vi "DataAcquisition.vi"() -> ()   [LabVIEW 2021]
uses:
  <instrlib>/niDMM/nidmm.llb/niDMM Function.ctl
  <instrlib>/niDMM/nidmm.llb/niDMM Configure Measurement Absolute.vi
  <instrlib>/niSwitch/niSwitch.llb/niSwitch Connect Channels (Single).vi
  <vilib>/express/express analysis/Spectral/Block/exnSpectralBlock spectral measurements RMS poly.vi
  <vilib>/express/express analysis/Spectral/Block/exnSpectralBlock spectral measurements RMS DDT.vi
  <vilib>/express/express analysis/Spectral/XNode/ExpressSpectralMeasurementsBlockNode.xnode
panel:
  out "Spectral Analysis: Magnitude":dynamicdata(graph)
  in  "Number Of Drops":dbl
  in  "Path":path
  out "2nd Trigger":bool
  out "1st Trigger":bool
  out "Spectral Analysis: Phase":dynamicdata(graph)
  out "Time Series":dynamicdata(graph)
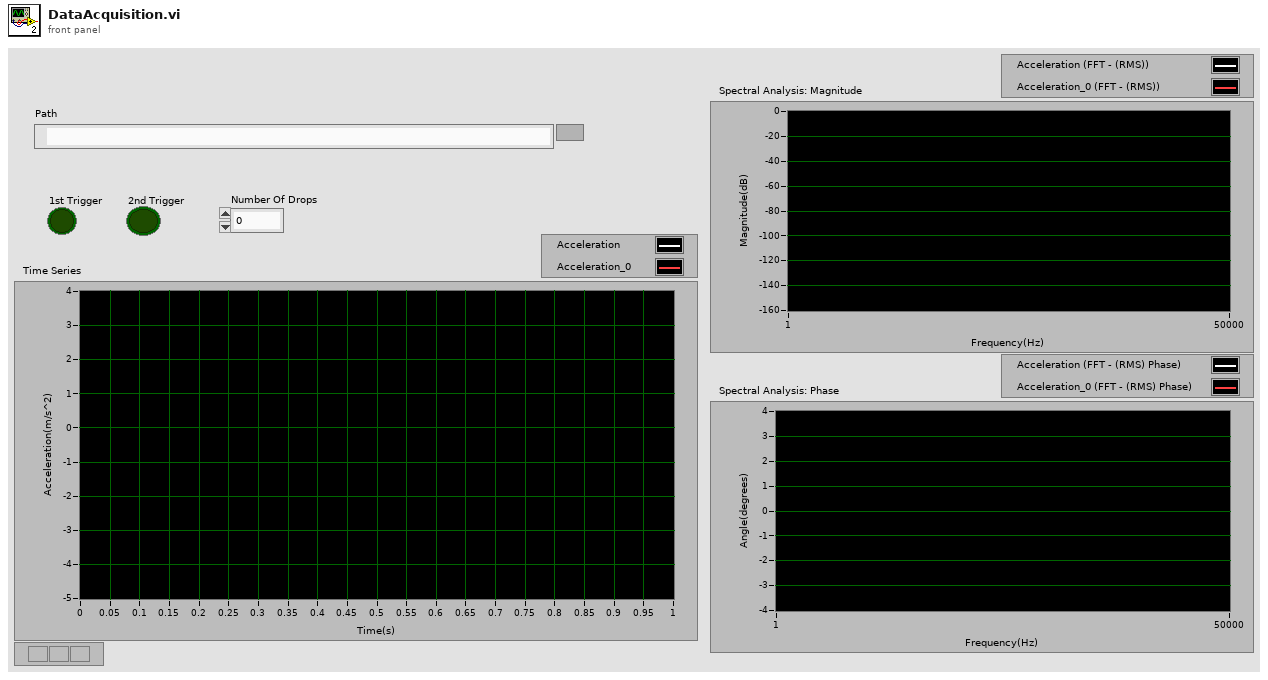
[diagram p1: front panel]
types:
  T1 = typedef "niDMM Function.ctl" = enum16{"DC Volts", "AC Volts", "DC Current", "AC Current", "2-wire Resistance", "4-wire Resistance", "Diode", "Frequency", "Period", "AC Volts DC Coupled", "Capacitance", "Inductance", "Temperature"}
  T2 = enum16{"open", "replace", "create", "open or create", "replace or create", "replace or create with confirmation"}
  T3 = cluster{"averaging mode":u16, "weighting mode":u16, "number of averages":u32}
  T4 = cluster{"dB On (F)":bool, "unwrap phase (F)":bool, "convert to degree (F)":bool}
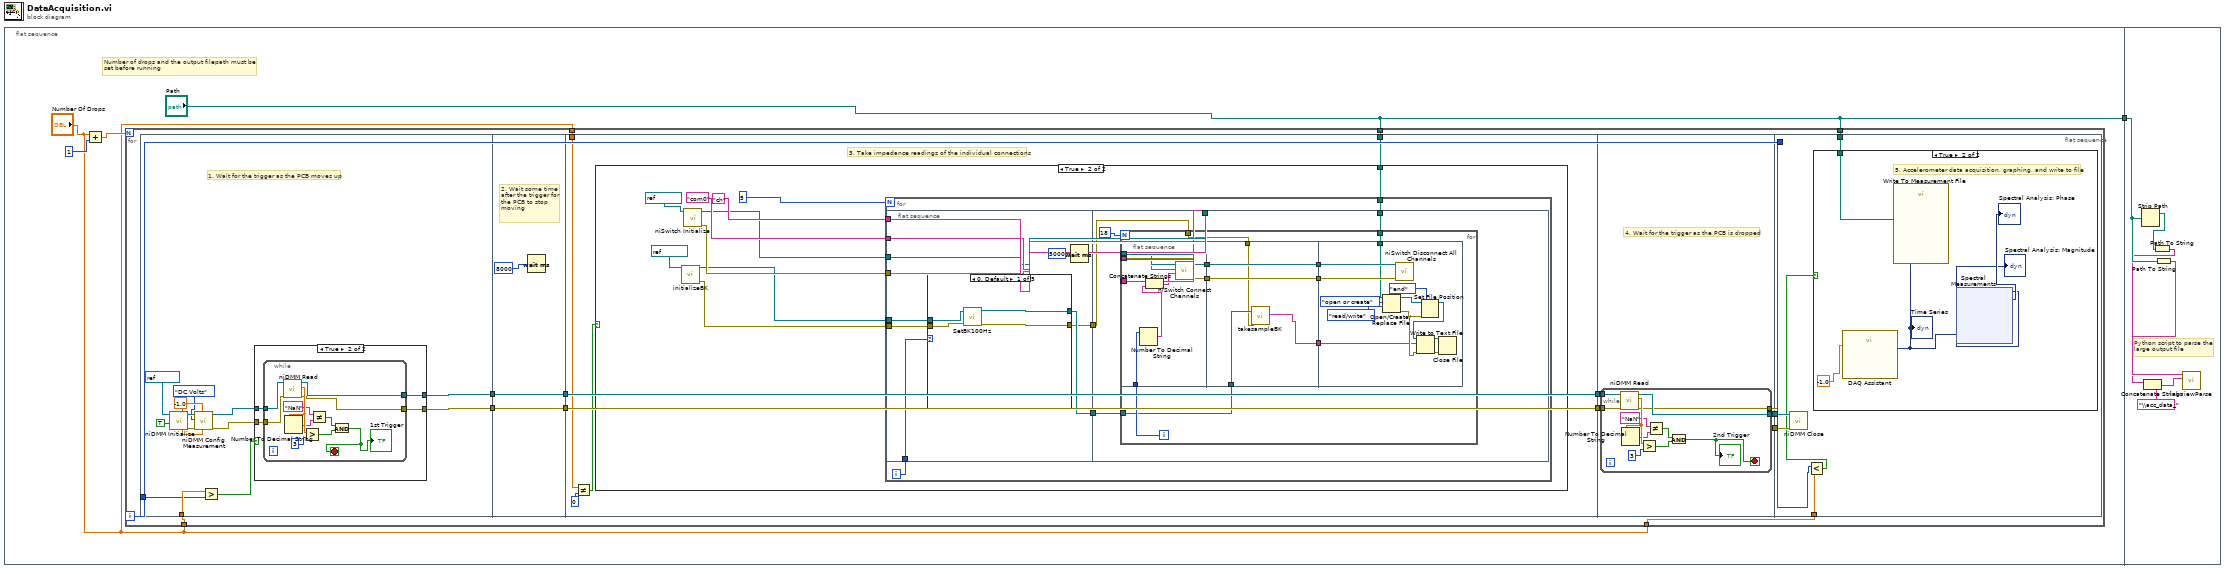
[diagram p0: block diagram]
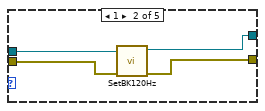
[diagram p4: hidden frame]
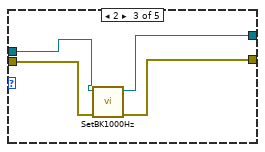
[diagram p5: hidden frame]
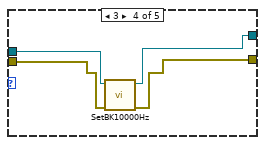
[diagram p6: hidden frame]
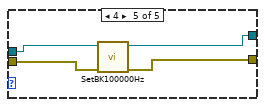
[diagram p7: hidden frame]
diagram:
  n1 = flat-sequence {
    tunnel: ["Path"] -> w1
    tunnel: w1 -> [w193]
    frame #0 {
      # "Number of drops and the output filepath must be\nset before running"
      n2 = Add(x="Number Of Drops", y=1) -> (x+y=w4:dbl)
      n3 = for {
        N: w4 -> [_]
        tunnel: "Number Of Drops" -> [w15]
        tunnel: "Number Of Drops" -> [w14]
        tunnel: "Path" -> [w8]
        tunnel: "Number Of Drops" -> [w7]
        tunnel: "Path" -> [w6]
        i -> [w13]
        n4 = flat-sequence {
          tunnel: [w24] -> w12
          tunnel: [w23] -> w10
          tunnel: w14 -> [w22]
          tunnel: w13 -> [w21]
          tunnel: w12 -> [w52]
          tunnel: [w52] -> w11
          tunnel: w10 -> [w51]
          tunnel: [w51] -> w9
          tunnel: [w58] -> w19
          tunnel: w11 -> [w58]
          tunnel: [w57] -> w18
          tunnel: w9 -> [w57]
          tunnel: w7 -> [w55]
          tunnel: w6 -> [w53]
          tunnel: w19 -> [w156]
          tunnel: w18 -> [w155]
          tunnel: [w154] -> w17
          tunnel: [w153] -> w16
          tunnel: w17 -> [w173]
          tunnel: w16 -> [w172]
          tunnel: w13 -> [w171]
          tunnel: w15 -> [w170]
          tunnel: w8 -> [w168]
          frame #0 {
            w27 = -1.0
            # "1. Wait for the trigger as the PCB moves up"
            n5 = call <instrlib>:"niDMM Initialize.vi"("Reset"=TRUE, "Instrument Descriptor"=refnum<k15> "DMM") -> ("error out"=w29:errorcluster, "instrument handle out"=w30:refnum<k15>)  [unwired: 8 in]
            n6 = call-poly <instrlib>:"niDMM Config Measurement.vi"("Range"=w27, "Resolution"=w27, "error in (no error)"=w29, "Function"=niDMM_Function."DC Volts", "instrument handle"=w30) -> ("error out"=w32:errorcluster, "instrument handle out"=w31:refnum<k15>)  [unwired: 5 in]
            n7 = Greater?(x=w22, y=w21) -> (0:w20:bool)
            n8 = case shown="True" w20 {
              tunnel: w32 -> [w34 w38]
              tunnel: w31 -> [w33 w37]
              tunnel: [w33 w36] -> w24
              tunnel: [w34 w35] -> w23
              frame False {
              }
              frame True {
                n9 = while {
                  tunnel: w37 -> [w49]
                  tunnel: w38 -> [w48]
                  tunnel: [w41] -> w36
                  tunnel: [w40] -> w35
                  stop <- w39 stop-if-true
                  n10 = call <instrlib>:"niDMM Read.vi"("error in (no error)"=w48, "instrument handle"=w49) -> ("error out"=w40:errorcluster, "Measurement"=w46:dbl, "instrument handle out"=w41:refnum<k15>)  [unwired: 7 in]
                  n11 = Number To Decimal String(number=w46) -> (decimal integer string=w44:string)  [unwired: 1 in]
                  n12 = Greater?(x=w46, y=3) -> (0:w42:bool)
                  n13 = Not Equal?(x="NaN", y=w44) -> (x != y?=w43:bool)
                  n14 = And(x=w43, y=w42) -> (x .and. y?=w39:bool)
                  "1st Trigger" <- w39
                }
              }
            }
          }
          frame #1 {
            # "2. Wait some time\nafter the trigger for the PCB to stop moving"
            n15 = Wait (ms)(milliseconds to wait=u32 8000) -> ()  [unwired: 1 out]
          }
          frame #2 {
            # "3. Take impedance readings of the individual connections"
            n16 = Not Equal?(x=w55, y=0) -> (x != y?=w54:bool)
            n17 = case shown="True" w54 {
              tunnel: w53 -> [_ w59]
              frame False {
              }
              frame True {
                n18 = call "initializeBK.vi"("VISA resource name"=refnum<visa-resource-name> "COM7") -> ("error out"=w60:errorcluster, "VISA resource name out"=w61:refnum<visa-resource-name>)  [unwired: 8 in, 1 out]
                n19 = call <instrlib>:"niSwitch Initialize.vi"("resource name"=refnum<k15> "switch") -> ("error out"=w64:errorcluster, "instrument handle out"=w63:refnum<k15>)  [unwired: 9 in]
                n20 = for {
                  N: 5 -> [_]
                  tunnel: "ch" -> [w79]
                  tunnel: "com0" -> [w78]
                  tunnel: w64 -> [w77]
                  tunnel: w63 -> [w76]
                  tunnel: w61 -> [w74]
                  tunnel: w60 -> [w73]
                  tunnel: w59 -> [w70]
                  i -> [w75]
                  n21 = flat-sequence {
                    tunnel: w75 -> [w84]
                    tunnel: w74 -> [w83]
                    tunnel: w73 -> [w82]
                    tunnel: [w81] -> w72
                    tunnel: [w80] -> w71
                    tunnel: w79 -> [w112]
                    tunnel: w78 -> [w111]
                    tunnel: w77 -> [w110]
                    tunnel: w76 -> [w109]
                    tunnel: w72 -> [w107]
                    tunnel: w71 -> [w106]
                    tunnel: w70 -> [w105]
                    frame #0 {
                      n22 = case shown="0, Default" w84 {
                        tunnel: w83 -> [w88 w92 w96 w100 w104]
                        tunnel: w82 -> [w87 w91 w95 w99 w101]
                        tunnel: [w86 w90 w93 w97 w103] -> w81
                        tunnel: [w85 w89 w94 w98 w102] -> w80
                        frame 0, Default {
                          n23 = call "SetBK100Hz.vi"("error out 2"=w87, "VISA resource name out"=w88) -> ("error out"=w85:errorcluster, "VISA resource name out 2"=w86:refnum<visa-resource-name>)  [unwired: 5 in]
                        }
                        frame 1 {
                          n24 = call "SetBK120Hz.vi"("error out 2"=w91, "VISA resource name out"=w92) -> ("error out"=w89:errorcluster, "VISA resource name out 2"=w90:refnum<visa-resource-name>)  [unwired: 8 in]
                        }
                        frame 2 {
                          n25 = call "SetBK1000Hz.vi"("VISA resource name out"=w96, "error out 2"=w95) -> ("VISA resource name out 2"=w93:refnum<visa-resource-name>, "error out"=w94:errorcluster)  [unwired: 7 in]
                        }
                        frame 3 {
                          n26 = call "SetBK10000Hz.vi"("VISA resource name out"=w100, "error out 2"=w99) -> ("VISA resource name out 2"=w97:refnum<visa-resource-name>, "error out"=w98:errorcluster)  [unwired: 6 in]
                        }
                        frame 4 {
                          n27 = call "SetBK100000Hz.vi"("error out 2"=w101, "VISA resource name out"=w104) -> ("error out"=w102:errorcluster, "VISA resource name out 2"=w103:refnum<visa-resource-name>)  [unwired: 8 in]
                        }
                      }
                    }
                    frame #1 {
                      n28 = for {
                        N: 18 -> [_]
                        tunnel: w112 -> [w120]
                        tunnel: w111 -> [w119]
                        tunnel: w110 -> [w118]
                        tunnel: w109 -> [w117]
                        tunnel: w107 -> [w116]
                        tunnel: w106 -> [w115]
                        tunnel: w105 -> [w113]
                        i -> [w121]
                        n29 = flat-sequence {
                          tunnel: w117 -> [w134]
                          tunnel: w118 -> [w133]
                          tunnel: w119 -> [w132]
                          tunnel: [w131] -> w124
                          tunnel: [w130] -> w122
                          tunnel: w121 -> [w129]
                          tunnel: w120 -> [w126]
                          tunnel: [w139] -> w125
                          tunnel: w124 -> [w139]
                          tunnel: [w138] -> w123
                          tunnel: w122 -> [w138]
                          tunnel: w116 -> [w137]
                          tunnel: w115 -> [w136]
                          tunnel: [w135] -> w114
                          tunnel: w125 -> [w152]
                          tunnel: w123 -> [w151]
                          tunnel: w114 -> [w146]
                          tunnel: w113 -> [w140]
                          frame #0 {
                            n30 = Number To Decimal String(number=w129) -> (decimal integer string=w127:string)  [unwired: 1 in]
                            n31 = Concatenate Strings(w126, w127) -> (w128:string)
                            n32 = call-poly <instrlib>:"niSwitch Connect Channels.vi"("error in (no error)"=w133, "channel 2"=w128, "channel 1"=w132, "instrument handle"=w134) -> ("error out"=w130:errorcluster, "instrument handle out"=w131:refnum<k15>)  [unwired: 6 in]
                          }
                          frame #1 {
                            n33 = call "takesampleBK.vi"("error in (no error)"=w136, "VISA resource name"=w137) -> ("current sample"=w135:string)  [unwired: 7 in, 2 out]
                          }
                          frame #2 {
                            n34 = Open/Create/Replace File(file path (use dialog)=w140, operation (0:open)=T2."open or create", access (0:read/write)=enum16{"read/write", "read-only", "write-only"}."read/write") -> (refnum out=w150:refnum<file>, error out=w149:errorcluster)  [unwired: 3 in, 1 out]
                            n35 = call <instrlib>:"niSwitch Disconnect All Channels.vi"("error in (no error)"=w151, "instrument handle"=w152) -> ()  [unwired: 8 in, 2 out]
                            n36 = Set File Position(refnum=w150, from (0:start)=enum16{"start", "end", "current"}."end", error in=w149) -> (refnum out=w148:refnum<file>, error out=w147:errorcluster)  [unwired: 1 in]
                            n37 = Write to Text File(file (use dialog)=w148, text=w146, error in=w147) -> (refnum out=w141:refnum<file>, error out=w142:errorcluster)  [unwired: 1 in, 1 out]
                            n38 = Close File(refnum=w141, error in=w142) -> ()  [unwired: 2 out]
                          }
                        }
                      }
                    }
                  }
                }
                n39 = Wait (ms)(milliseconds to wait=u32 5000) -> ()  [unwired: 1 out]
              }
            }
          }
          frame #3 {
            # "4. Wait for the trigger as the PCB is dropped"
            n40 = while {
              tunnel: w156 -> [w161]
              tunnel: w155 -> [w160]
              tunnel: [w159] -> w154
              tunnel: [w158] -> w153
              stop <- w157 stop-if-true
              n41 = call <instrlib>:"niDMM Read.vi"("error in (no error)"=w160, "instrument handle"=w161) -> ("error out"=w158:errorcluster, "Measurement"=w166:dbl, "instrument handle out"=w159:refnum<k15>)  [unwired: 7 in]
              n42 = Number To Decimal String(number=w166) -> (decimal integer string=w164:string)  [unwired: 1 in]
              n43 = Greater?(x=w166, y=3) -> (0:w162:bool)
              n44 = Not Equal?(x="NaN", y=w164) -> (x != y?=w163:bool)
              n45 = And(x=w163, y=w162) -> (x .and. y?=w157:bool)
              "2nd Trigger" <- w157
            }
          }
          frame #4 {
            n46 = call <instrlib>:"niDMM Close.vi"("error in (no error)"=w172, "instrument handle"=w173) -> ()  [unwired: 9 in, 1 out]
            n47 = Less?(x=w171, y=w170) -> (x < y?=w169:bool)
            n48 = case shown="True" w169 {
              tunnel: w168 -> [_ w174]
              frame False {
              }
              frame True {
                # "5. Accelerometer data acquisition, graphing, and write to file"
                n49 = call "DAQ Assistant"("timeout (s)"=-1.0) -> ("data"=w177:dynamicdata)  [unwired: 16 in, 2 out]
                "Time Series" <- w177
                n50 = call "Write To Measurement File"("Signals"=w177, "Filename"=w174) -> ()  [unwired: 15 in, 3 out]
                n51 = xnode "Spectral Measurements"("Signals"=w177) -> ("FFT - (RMS)"=→"Spectral Analysis: Magnitude":dynamicdata, "Phase"=→"Spectral Analysis: Phase":dynamicdata)  [unwired: 1 in, 1 out]
              }
            }
          }
        }
      }
    }
    frame #1 {
      # "Python script to parse the\nlarge output file"
      n52 = Strip Path(path=w193) -> (stripped path=w194:path)  [unwired: 1 out]
      n53 = Path To String(path=w194) -> (string=w191:string)
      n54 = Concatenate Strings(w191, "\\acc_data_") -> (w189:string)
      n55 = Path To String(path=w193) -> (string=w192:string)
      n56 = call "labviewParse.vi"("outFolderPath"=w189, "InFilePath"=w192) -> ()  [unwired: 10 in]
    }
  }
